vi "Wait_Seconds_with_display.vi"(2 "Message":string, 3 "Seconds to wait":dbl=1.0 format="%.2f") -> (1 "Stopped":bool)   [LabVIEW 2010]
doc: "Waits the number of seconds specified by the Seconds to Wait input, divided by the time dilation factor, if used."
panel:
  in  "stop":bool
  out "Seconds waited":u32(slide) scale=0.0..5.0
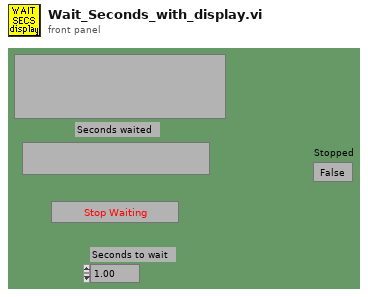
[diagram p1: front panel]
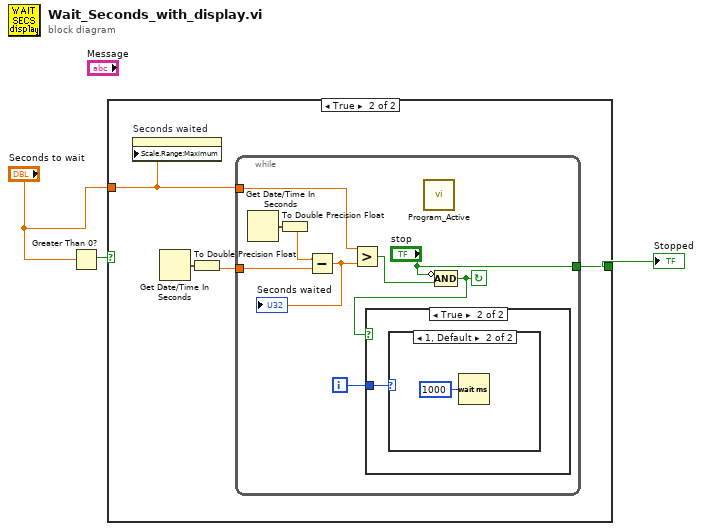
[diagram p0: block diagram]
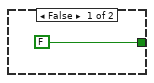
[diagram p2: hidden frame]
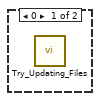
[diagram p4: hidden frame]
diagram:
  n1 = Greater Than 0?(x="Seconds to wait") -> (x > 0?=w2:bool)
  n2 = case shown="True" w2 {
    tunnel: [FALSE ("stop") w8] -> w3
    tunnel: "Seconds to wait" -> [_ w6]
    frame False {
    }
    frame True {
      n3 = property on="Seconds waited" class="Slide (strict)"("Scale.Range:Maximum"=w6) -> ()  [unwired: 2 in, 2 out]
      n4 = Get Date/Time In Seconds() -> (seconds since 1Jan1904=w5:timestamp)
      n5 = To Double Precision Float(number=w5) -> (double precision float=w7:dbl)
      n6 = while {
        tunnel: ["stop"] -> w8
        tunnel: w6 -> [w14]
        tunnel: w7 -> [w17]
        i -> [w9]
        stop <- w10 continue-if-true
        n7 = Get Date/Time In Seconds() -> (seconds since 1Jan1904=w11:timestamp)
        n8 = To Double Precision Float(number=w11) -> (double precision float=w12:dbl)
        n9 = Subtract(x=w12, y=w17) -> (x-y=w13:dbl)
        "Seconds waited" <- w13
        n10 = Greater?(x=w14, y=w13) -> (0:w16:bool)
        n11 = call "Program_Active.vi"() -> ()  [unwired: 1 in]
        n12 = Compound Arithmetic op=AND(invert "stop", w16) -> (w10:bool)
        n13 = case shown="True" w10 {
          tunnel: w9 -> [_ w18]
          frame False {
          }
          frame True {
            n14 = case shown="1, Default" w18 {
              frame 0 {
                n15 = call "Try_Updating_Files.vi"() -> ()  [unwired: 4 out]
              }
              frame 1, Default {
                n16 = Wait (ms)(milliseconds to wait=u32 1000) -> ()  [unwired: 1 out]
              }
            }
          }
        }
      }
    }
  }
  "Stopped" <- w3
